vi "Move Step.vi"(10 "Move Down?":bool, 11 "Settings UI in":refnum<class "Settings UI.lvclass">) -> (3 "Settings UI out":refnum<class "Settings UI.lvclass">)   [LabVIEW 2020, in "Output Sequencer.lvlib" / "Settings UI.lvclass"]
uses:
  Settings UI.lvclass
  Settings UI.lvclass/Settings UI.ctl
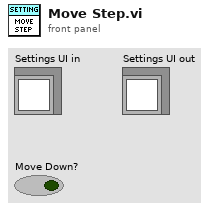
[diagram p1: front panel]
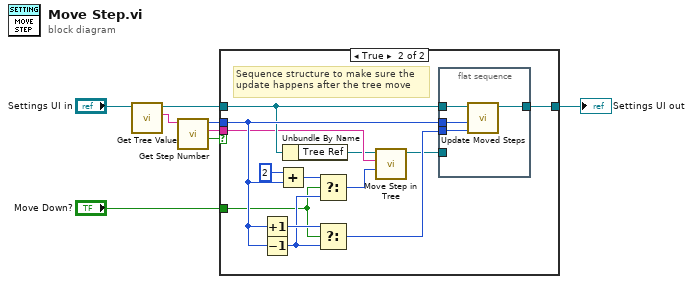
[diagram p0: block diagram]
diagram:
  n1 = call "Get Tree Value.vi"("UI Data in"="Settings UI in") -> ("Value"=w3:string, "UI Data out"=w6:refnum<class "Settings UI.lvclass">)  [unwired: 9 in]
  n2 = call "Get Step Number.vi"("Tree Tag"=w3) -> ("Is Step tag?"=w4:bool, "Step tag"=w5:string, "Step Number"=w2:i32)  [unwired: 8 in]
  n3 = case shown="True" w4 {
    tunnel: w2 -> [_ w17]
    tunnel: w6 -> [w9 w14]
    tunnel: [w9 w16] -> w7
    tunnel: w5 -> [_ w12]
    tunnel: "Move Down?" -> [_ w15]
    frame False {
    }
    frame True {
      # "Sequence structure to make sure the\nupdate happens after the tree move"
      n4 = Increment(x=w17) -> (x+1=w20:i32)
      n5 = Decrement(x=w17) -> (x-1=w19:i32)
      n6 = Add(x=2, y=w17) -> (x+y=w21:i32)
      n7 = Unbundle By Name(w14) -> ("Tree Ref"=w10:refnum<vi>)
      n8 = Select(t=w21, s=w15, f=w19) -> (s? t:f=w11:i32)
      n9 = Select(t=w20, s=w15, f=w19) -> (s? t:f=w18:i32)
      n10 = call "Move Step in Tree.vi"("New Position"=w11, "Step Tag"=w12, "TreeControl in"=w10) -> ("TreeControl out"=w13:refnum<vi>)  [unwired: 8 in]
      n11 = flat-sequence {
        tunnel: w18 -> [w26]
        tunnel: w17 -> [w25]
        tunnel: w14 -> [w24]
        tunnel: [w23] -> w16
        tunnel: w13 -> [_]
        frame #0 {
          n12 = call "Update Moved Steps.vi"("New Step Number"=w26, "Previous Step Number"=w25, "UI Data In"=w24) -> ("UI Data Out"=w23:refnum<class "Settings UI.lvclass">)  [unwired: 8 in]
        }
      }
    }
  }
  "Settings UI out" <- w7
